vi "Update Shield.vi"(11 "Board Game in":refnum<class "Board Game.lvclass">) -> ()   [LabVIEW 2021, in "Board Game.lvclass"]
uses:
  Board Game.lvclass
  Board Game.lvclass/Board Game.ctl
  Shield/Shield.lvclass/Shield.ctl
  Application/Shield.ctl
  Shield/Read Shield Count.vi
  Application/Game.lvclass
  Shield/Shield.lvclass
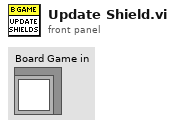
[diagram p1: front panel]
types:
  T1 = typedef "Game.lvclass/Shield.ctl" = u16
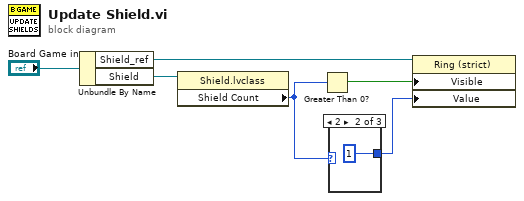
[diagram p0: block diagram]
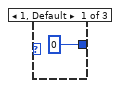
[diagram p2: hidden frame]
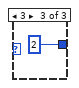
[diagram p3: hidden frame]
diagram:
  n1 = Unbundle By Name("Board Game in") -> ("Shield_ref"=w3:refnum<vi>, "Shield"=w2:refnum<class "Shield.lvclass">)
  n2 = property class="Shield.lvclass"(reference=w2) -> ("Shield Count"=w5:u8)  [unwired: 1 in, 2 out]
  n3 = Greater Than 0?(x=w5) -> (x > 0?=w4:bool)
  n4 = case shown="2" w5 {
    tunnel: [T1 0 ("Value") T1 1 ("Value") T1 2 ("Value")] -> w6
    frame 1, Default {
    }
    frame 2 {
    }
    frame 3 {
    }
  }
  n5 = property class="Ring (strict)"(reference=w3, "Visible"=w4, "Value"=w6) -> ()  [unwired: 1 in, 2 out]
